vi "App_Open Image.vi"(8 "error in":errorcluster, 11 "Image":T1) -> (0 "error out":errorcluster)   [LabVIEW 2015, in "Application 1.lvlib"]
uses:
  Application 1.lvlib
  <vilib>/vision/Image Controls.llb/IMAQ Image.ctl
  <vilib>/vision/NI_Vision_Development_Module.lvlib
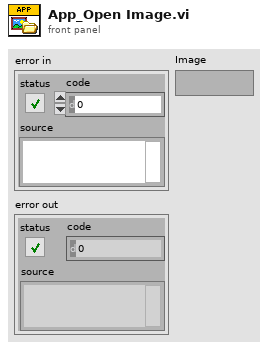
[diagram p1: front panel]
types:
  T1 = typedef "IMAQ Image.ctl" = refnum<image>
  T2 = typedef "Image Type" = u32
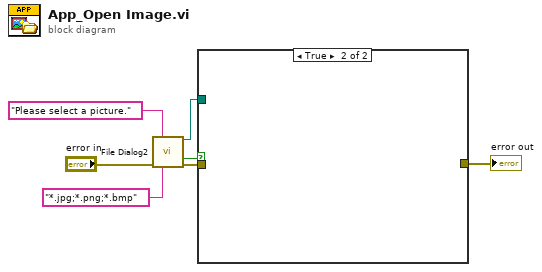
[diagram p0: block diagram]
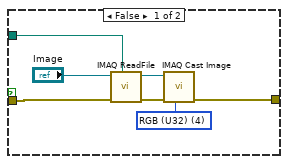
[diagram p2: hidden frame]
diagram:
  n1 = call "File Dialog2"("prompt"="Please select a picture.", "error in"="error in", "pattern (all files)"="*.jpg;*.png;*.bmp") -> ("selected path"=w3:path, "cancelled"=w5:bool, "error out"=w4:errorcluster)  [unwired: 9 in, 1 out]
  n2 = case shown="True" w5 {
    tunnel: w4 -> [w14 _]
    tunnel: w3 -> [w13 _]
    tunnel: [w8 _] -> w1
    frame False {
      w9 = T2 4 items=["Grayscale (U8)", "Grayscale (I16)", "Grayscale (SGL)", "Complex (CSG)", "RGB (U32)", "HSL (U32)", "RGB (U64)", "Grayscale (U16)"] ("Image Type")
      n3 = call "IMAQ ReadFile"("File Path"=w13, "error in (no error)"=w14, "Image"="Image") -> ("error out"=w11:errorcluster, "Image Out"=w10:T1)  [unwired: 4 in, 3 out]
      n4 = call "IMAQ Cast Image"("Image Type"=w9, "error in (no error)"=w11, "Image Src"=w10) -> ("error out"=w8:errorcluster)  [unwired: 7 in, 1 out]
    }
    frame True {
    }
  }
  "error out" <- w1
